vi "tcpMessageServer.vi"(11 "server configuration":T1={"client ID"="tcpServer", "remote host"="", "local port"=50001, "remote port"=0}) -> (0 "error out":errorcluster)   [LabVIEW 2014]
doc: "A couple tcpMessageServer and tcpMessageClient ensures communication between two instances. Each one can both transmit or receive CR/LF terminated message strings; however one of the member has to be a Server and the other a Client. Both sit and wait for the other party to connect.\n\nThe difference is: \n* the Server accpts connections on the specified port from any incoming host (the inputs \"remote host\" and \"remote port\" are ignored) \n* the Client must know to which host is directed\n\nCommunication with them, while running, is done via four named queues. One acts as a transmission buffer, another as a receive buffer; one is a single element queue, which cause the shutdown of the actor when a True is enqueued to it; the last one is a read only one-element queue which reports the actor status."
uses:
  typedefs/clientStatus.ctl
  typedefs/clientConfiguration.ctl
panel:
  out "remote address":string
  out "remote port":u16
  out "string to send":string
  out "received string":string
  out "status":T2
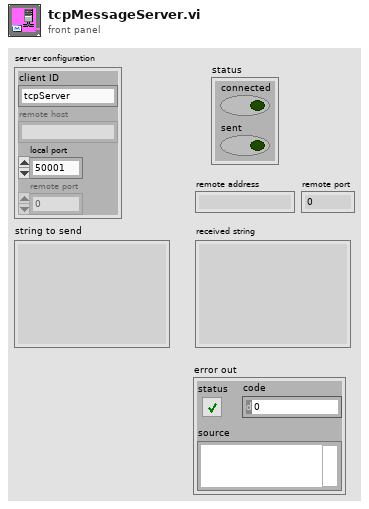
[diagram p1: front panel]
types:
  T1 = typedef "clientConfiguration.ctl" = cluster{"client ID":string, "remote host":string, "local port":u16, "remote port":u16}
  T2 = typedef "clientStatus.ctl" = cluster{"connected":bool, "sent":bool}
  T3 = cluster{"status":cluster{"queue":refnum<queue>, "error out":errorcluster}, "receive":cluster{"queue":refnum<queue>, "error out":errorcluster}, "transmit":cluster{"queue":refnum<queue>, "error out":errorcluster}, "shutdown":cluster{"queue":refnum<queue>, "error out":errorcluster}}
  T4 = cluster{"queue":refnum<queue>, "error out":errorcluster}
  T5 = enum16{"Standard", "Buffered", "CRLF", "Immediate"}
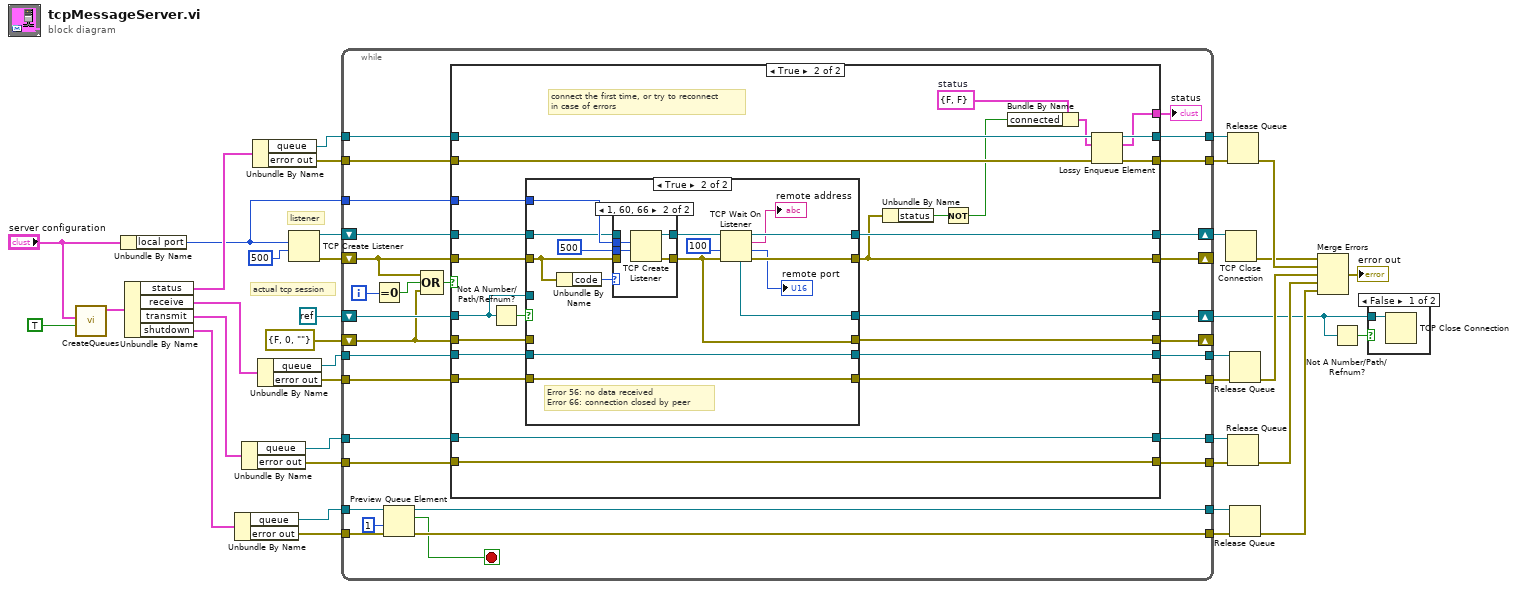
[diagram p0: block diagram]
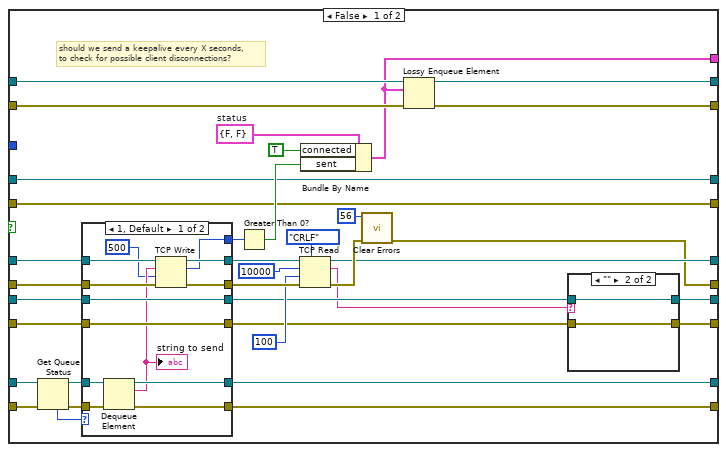
[diagram p3: hidden frame]
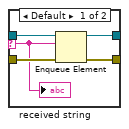
[diagram p4: hidden frame]
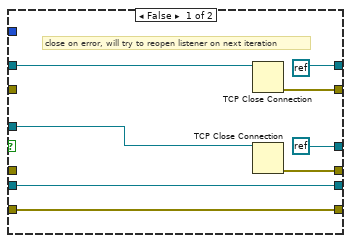
[diagram p6: hidden frame]
diagram:
  # "listener"
  # "actual tcp session"
  n1 = call "CreateQueues.vi"("create if not found? (T)"=TRUE, "client configuration"="server configuration") -> ("output cluster"=w2:T3)  [unwired: 9 in]
  n2 = Unbundle By Name("server configuration") -> ("local port"=w7:u16)
  n3 = Unbundle By Name(w2) -> ("status"=w36:T4, "receive"=w33:T4, "transmit"=w32:T4, "shutdown"=w27:T4)
  n4 = Unbundle By Name(w27) -> ("queue"=w28:refnum<queue>, "error out"=w29:errorcluster)
  n5 = Unbundle By Name(w32) -> ("queue"=w31:refnum<queue>, "error out"=w30:errorcluster)
  n6 = Unbundle By Name(w36) -> ("queue"=w37:refnum<queue>, "error out"=w38:errorcluster)
  n7 = Unbundle By Name(w33) -> ("queue"=w34:refnum<queue>, "error out"=w35:errorcluster)
  n8 = TCP Create Listener(9:500 ("timeout ms (25000)"), 10:w7) -> (0:w10:errorcluster, 3:w11:refnum<k5>)  [unwired: 3 in, 1 out]
  n9 = while {
    shift-right: [w67] -> _
    shift-left: w10 -> [w66]
    shift-right: [w68] -> w12
    shift-left: w11 -> [w69]
    tunnel: w29 -> [w44]
    tunnel: w28 -> [w45]
    tunnel: w37 -> [w62]
    tunnel: w38 -> [w61]
    tunnel: w34 -> [w60]
    tunnel: w35 -> [w59]
    tunnel: w31 -> [w58]
    tunnel: w30 -> [w57]
    tunnel: [w43] -> w13
    tunnel: [w42] -> w14
    tunnel: [w56] -> w15
    tunnel: [w55] -> w16
    tunnel: [w53] -> w17
    tunnel: [w52] -> w18
    tunnel: [w51] -> w19
    tunnel: [w50] -> w20
    shift-right: [w47] -> w5
    shift-left: refnum<k0> refnum -> [w48]
    tunnel: w7 -> [w49]
    shift-right: [w46] -> _
    shift-left: errorcluster {"status"=FALSE, "code"=0, "source"=""} ("error out") -> [w39]
    i -> [w65]
    stop <- w41 stop-if-true
    n10 = Equal To 0?(x=w65) -> (x = 0?=w64:bool)
    n11 = Preview Queue Element(queue=w45, timeout in ms (-1)=1, error in (no error)=w44) -> (queue out=w43:refnum<queue>, element=w41:bool, error out=w42:errorcluster)  [unwired: 1 out]
    n12 = Compound Arithmetic op=OR(w66, w64, w39) -> (w63:bool)
    n13 = case shown="True" w63 {
      tunnel: w69 -> [w72 w146]
      tunnel: [w72 w143] -> w68
      tunnel: [w71 w136] -> w67
      tunnel: w66 -> [w71 w147]
      tunnel: w62 -> [w105 w155]
      tunnel: w61 -> [w104 w154]
      tunnel: w60 -> [w91 w142]
      tunnel: w59 -> [w90 w141]
      tunnel: w58 -> [w99 w151]
      tunnel: w57 -> [w98 w150]
      tunnel: [w103 w153] -> w56
      tunnel: [w102 w152] -> w55
      tunnel: [w94 w134] -> w54
      tunnel: [w80 w140] -> w53
      tunnel: [w79 w139] -> w52
      tunnel: [w93 w151] -> w51
      tunnel: [w92 w150] -> w50
      tunnel: w49 -> [_ w148]
      tunnel: w48 -> [w77 w145]
      tunnel: [w75 w144] -> w47
      tunnel: w39 -> [w76 w138]
      tunnel: [w73 w137] -> w46
      frame False {
        w101 = T2 {"connected"=FALSE, "sent"=FALSE}  # status
        # "should we send a keepalive every X seconds,\nto check for possible client disconnections?"
        n14 = Get Queue Status(queue=w99, error in (no error)=w98) -> (queue out=w96:refnum<queue>, error out=w95:errorcluster, # elements in queue=w97:i32)  [unwired: 1 in, 5 out]
        n15 = case shown="1, Default" w97 {
          tunnel: w96 -> [w125 w127]
          tunnel: w95 -> [w124 w126]
          tunnel: [w123 w127] -> w93
          tunnel: [w122 w126] -> w92
          tunnel: w91 -> [w121 w131]
          tunnel: w90 -> [w120 w130]
          tunnel: [w121 w131] -> w82
          tunnel: [w120 w130] -> w81
          tunnel: w77 -> [w119 w129]
          tunnel: w76 -> [w118 w128]
          tunnel: [w117 w129] -> w89
          tunnel: [w116 w128] -> w86
          tunnel: [w115 _] -> w88
          frame 1, Default {
            n16 = Dequeue Element(queue=w125, error in (no error)=w124) -> (queue out=w123:refnum<queue>, element=w114:string, error out=w122:errorcluster)  [unwired: 1 in, 1 out]
            "string to send" <- w114
            n17 = TCP Write(connection ID=w119, data in=w114, error in (no error)=w118, 9:500 ("timeout ms (25000)")) -> (connection ID out=w117:refnum<k5>, bytes written=w115:i32, error out=w116:errorcluster)
          }
          frame 0 {
          }
        }
        n18 = Greater Than 0?(x=w88) -> (x > 0?=w87:bool)
        n19 = TCP Read(connection ID=w89, bytes to read=10000, error in (no error)=w86, 7:T5."CRLF" ("mode (standard)"), 9:100 ("timeout ms (25000)")) -> (connection ID out=w75:refnum<k5>, data out=w78:string, error out=w85:errorcluster)
        n20 = Bundle By Name(cluster=w101, "connected"=TRUE, "sent"=w87) -> (w94:T2)
        n21 = call <vilib>:"Clear Errors.vi"("error in (no error)"=w85, "specific error code to clear (0: all)"=56) -> ("error out"=w73:errorcluster)  [unwired: 4 in, 1 out]
        n22 = Lossy Enqueue Element(queue=w105, element=w94, error in (no error)=w104) -> (queue out=w103:refnum<queue>, error out=w102:errorcluster)  [unwired: 2 out]
        n23 = case shown="\"\"" w78 {
          selector: w78 -> [w106 _]
          tunnel: w82 -> [w108 w112]
          tunnel: w81 -> [w107 w111]
          tunnel: [w110 w112] -> w80
          tunnel: [w109 w111] -> w79
          frame Default {
            n24 = Enqueue Element(queue=w108, element=w106, error in (no error)=w107) -> (queue out=w110:refnum<queue>, error out=w109:errorcluster)  [unwired: 1 in, 1 out]
            "received string" <- w106
          }
          frame "" {
          }
        }
      }
      frame True {
        w135 = T2 {"connected"=FALSE, "sent"=FALSE}  # status
        # "connect the first time, or try to reconnect\nin case of errors"
        n25 = Not A Number/Path/Refnum?(number/path/refnum=w145) -> (NaN/Path/Refnum?=w149:bool)
        n26 = case shown="True" w149 {
          tunnel: w146 -> [w161 w170]
          tunnel: w147 -> [_ w169]
          tunnel: [refnum<k0> refnum w178] -> w143
          tunnel: [w157 w176] -> w136
          tunnel: [refnum<k0> refnum w174] -> w144
          tunnel: w145 -> [w163 _]
          tunnel: w148 -> [_ w172]
          tunnel: w142 -> [w159 w168]
          tunnel: w141 -> [w158 w167]
          tunnel: [w159 w168] -> w140
          tunnel: [w158 w167] -> w139
          tunnel: w138 -> [_ _]
          tunnel: [w156 w164] -> w137
          frame False {
            # "close on error, will try to reopen listener on next iteration"
            n27 = TCP Close Connection(connection ID=w161) -> (error out=w157:errorcluster)  [unwired: 2 in, 1 out]
            n28 = TCP Close Connection(connection ID=w163) -> (error out=w156:errorcluster)  [unwired: 2 in, 1 out]
          }
          frame True {
            # "Error 56: no data received\nError 66: connection closed by peer"
            n29 = Unbundle By Name(w169) -> ("code"=w173:i32)
            n30 = case shown="1, 60, 66" w173 {
              tunnel: w172 -> [_ w183]
              tunnel: [w179 w182] -> w171
              tunnel: w170 -> [w179 _]
              tunnel: [_ w181] -> w164
              tunnel: w169 -> [_ _]
              tunnel: 500 -> [_ w180]
              frame 0, Default {
              }
              frame 1, 60, 66 {
                n31 = TCP Create Listener(9:w180, 10:w183) -> (0:w181:errorcluster, 3:w182:refnum<k5>)  [unwired: 3 in, 1 out]
              }
            }
            n32 = TCP Wait On Listener(8:w164, 9:100, 11:w171) -> (0:w176:errorcluster, 1:→"remote port":u16, 2:→"remote address":string, 3:w178:refnum<k5>, 4:w174:refnum<k5>)  [unwired: 1 in]
          }
        }
        n33 = Unbundle By Name(w136) -> ("status"=w133:bool)
        n34 = Not(x=w133) -> (.not. x?=w132:bool)
        n35 = Bundle By Name(cluster=w135, "connected"=w132) -> (w134:T2)
        n36 = Lossy Enqueue Element(queue=w155, element=w134, error in (no error)=w154) -> (queue out=w153:refnum<queue>, error out=w152:errorcluster)  [unwired: 2 out]
      }
    }
    "status" <- w54
  }
  n37 = TCP Close Connection(connection ID=w12) -> (error out=w21:errorcluster)  [unwired: 2 in, 1 out]
  n38 = Release Queue(queue=w15, error in (no error)=w16) -> (error out=w22:errorcluster)  [unwired: 1 in, 2 out]
  n39 = Release Queue(queue=w19, error in (no error)=w20) -> (error out=w24:errorcluster)  [unwired: 1 in, 2 out]
  n40 = Release Queue(queue=w17, error in (no error)=w18) -> (error out=w23:errorcluster)  [unwired: 1 in, 2 out]
  n41 = Release Queue(queue=w13, error in (no error)=w14) -> (error out=w25:errorcluster)  [unwired: 1 in, 2 out]
  n42 = Merge Errors(w21, w22, w23, w24, w25) -> (→"error out":errorcluster)
  n43 = Not A Number/Path/Refnum?(number/path/refnum=w5) -> (NaN/Path/Refnum?=w6:bool)
  n44 = case shown="False" w6 {
    tunnel: w5 -> [w184 _]
    frame False {
      n45 = TCP Close Connection(connection ID=w184) -> ()  [unwired: 2 in, 2 out]
    }
    frame True {
    }
  }
